vi "AnglesFromBinary.vi"(8 "Binary Offset":bool[][](array[boolean]), 10 "Array":bool[][](array[boolean]), 11 "Buffer Length":i32) -> (3 "Unwrapped Phase":dbl[][](array[numeric]))   [LabVIEW 2021]
uses:
  <vilib>/Analysis/NI_AALPro.lvlib
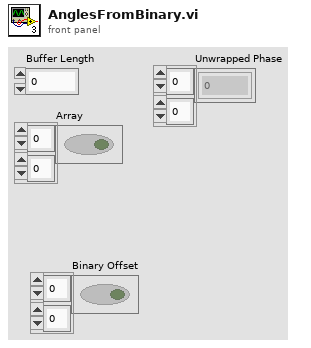
[diagram p1: front panel]
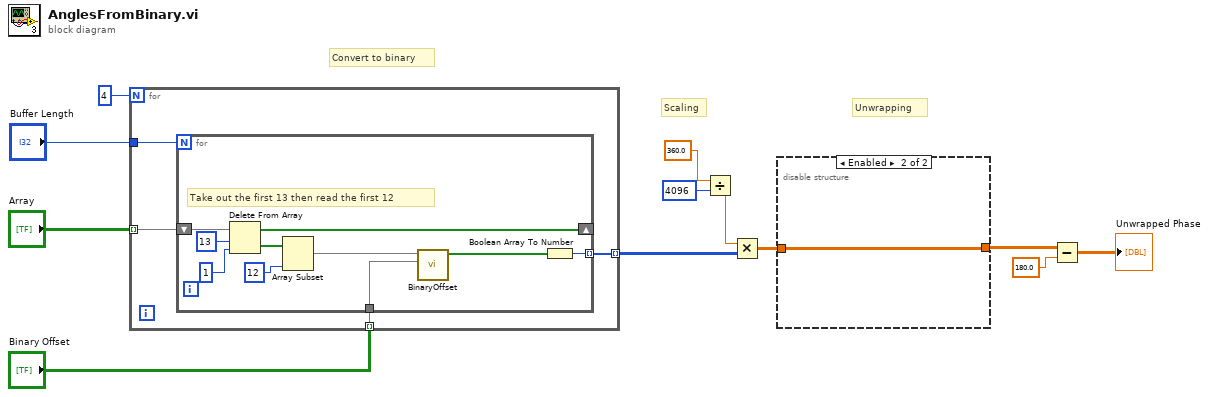
[diagram p0: block diagram]
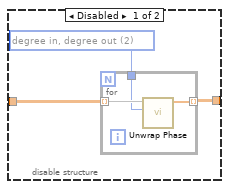
[diagram p2: hidden frame]
diagram:
  # "Unwrapping"
  # "Scaling"
  # "Convert to binary"
  n1 = for {
    N: 4 -> [_]
    tunnel: "Array" -> [w15] mode=indexing
    tunnel: [w16] -> w6 mode=indexing
    tunnel: "Buffer Length" -> [w14]
    tunnel: "Binary Offset" -> [w13] mode=indexing
    n2 = for {
      N: w14 -> [_]
      tunnel: [w26] -> w16 mode=indexing
      shift-right: [w25] -> _
      shift-left: w15 -> [w22]
      tunnel: w13 -> [w17]
      # "Take out the first 13 then read the first 12"
      n3 = Delete From Array(array=w22, length=13, index=1) -> (deleted portion=w19:bool[], array with subset deleted=w25:bool[])
      n4 = Array Subset(array=w19, length=12) -> (w20:bool[])  [unwired: 1 in]
      n5 = call "BinaryOffset.vi"("Offset in"=w17, "Number in"=w20) -> ("Array out"=w21:bool[])  [unwired: 9 in]
      n6 = Boolean Array To Number(Boolean array=w21) -> (number=w26:u32)
    }
  }
  n7 = Divide(x=360.0, y=4096) -> (x/y=w10:dbl)
  n8 = Multiply(x=w10, y=w6) -> (x*y=w5:dbl[][])
  n9 = disable-structure shown="Enabled" {
    disable-tunnel: w5 -> [w29 w33]
    disable-tunnel: [w28 w33] -> w3
    frame Disabled {
      w27 = 2 items=["radian in, radian out", "radian in, degree out", "degree in, degree out", "degree in, radian out"] ("phase unit")
      n10 = for {
        tunnel: [w32] -> w28 mode=indexing
        tunnel: w29 -> [w31] mode=indexing
        tunnel: w27 -> [w30]
        n11 = call <vilib>:"Unwrap Phase.vi"("phase unit"=w30, "Phase"=w31) -> ("Unwrapped Phase"=w32:dbl[])  [unwired: 8 in, 1 out]
      }
    }
    frame Enabled {
    }
  }
  n12 = Subtract(x=w3, y=180.0) -> (x-y=→"Unwrapped Phase":dbl[][])
